vi "CreateStringParams(SubVI).vi"(1 "Show Code":bool, 2 "Line Color":string, 3 "Autoscale Mode String":string, 4 "Line Number":dbl, 5 "Cluster Graph App":T2={"Min2"=0.0, "Name2"="", "Max2"=1.0, "Min"=0.0, "Name"="", "Max"=1.0}, 6 "Cluster Line Data":T1, 7 "Cluster Mode":T3) -> (0 "params":string)   [LabVIEW 2018]
panel:
  in  "Control":string
  # "Axis Y"
  # "Axis X"
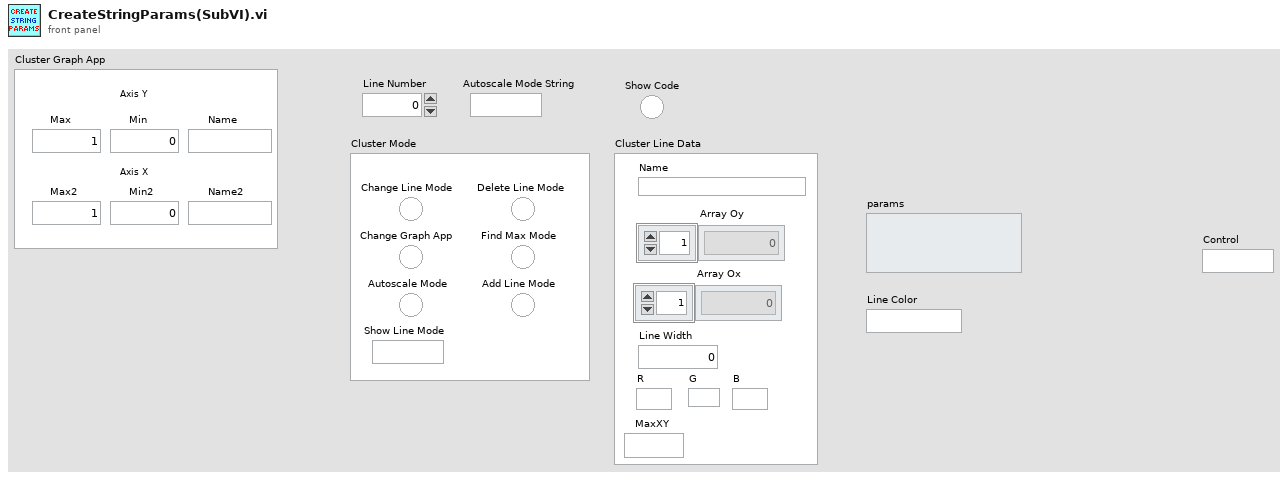
[diagram p1: front panel]
types:
  T1 = cluster{"Array Oy":dbl[], "Line Width":dbl, "Name":string, "R":string, "G":string, "B":string, "Array Ox":dbl[], "MaxXY":string}
  T2 = cluster{"Min2":dbl, "Name2":string, "Max2":dbl, "Min":dbl, "Name":string, "Max":dbl}
  T3 = cluster{"Change Line Mode":bool, "Delete Line Mode":bool, "Add Line Mode":bool, "Change Graph App":bool, "Autoscale Mode":bool, "Find Max Mode":bool, "Show Line Mode":string}
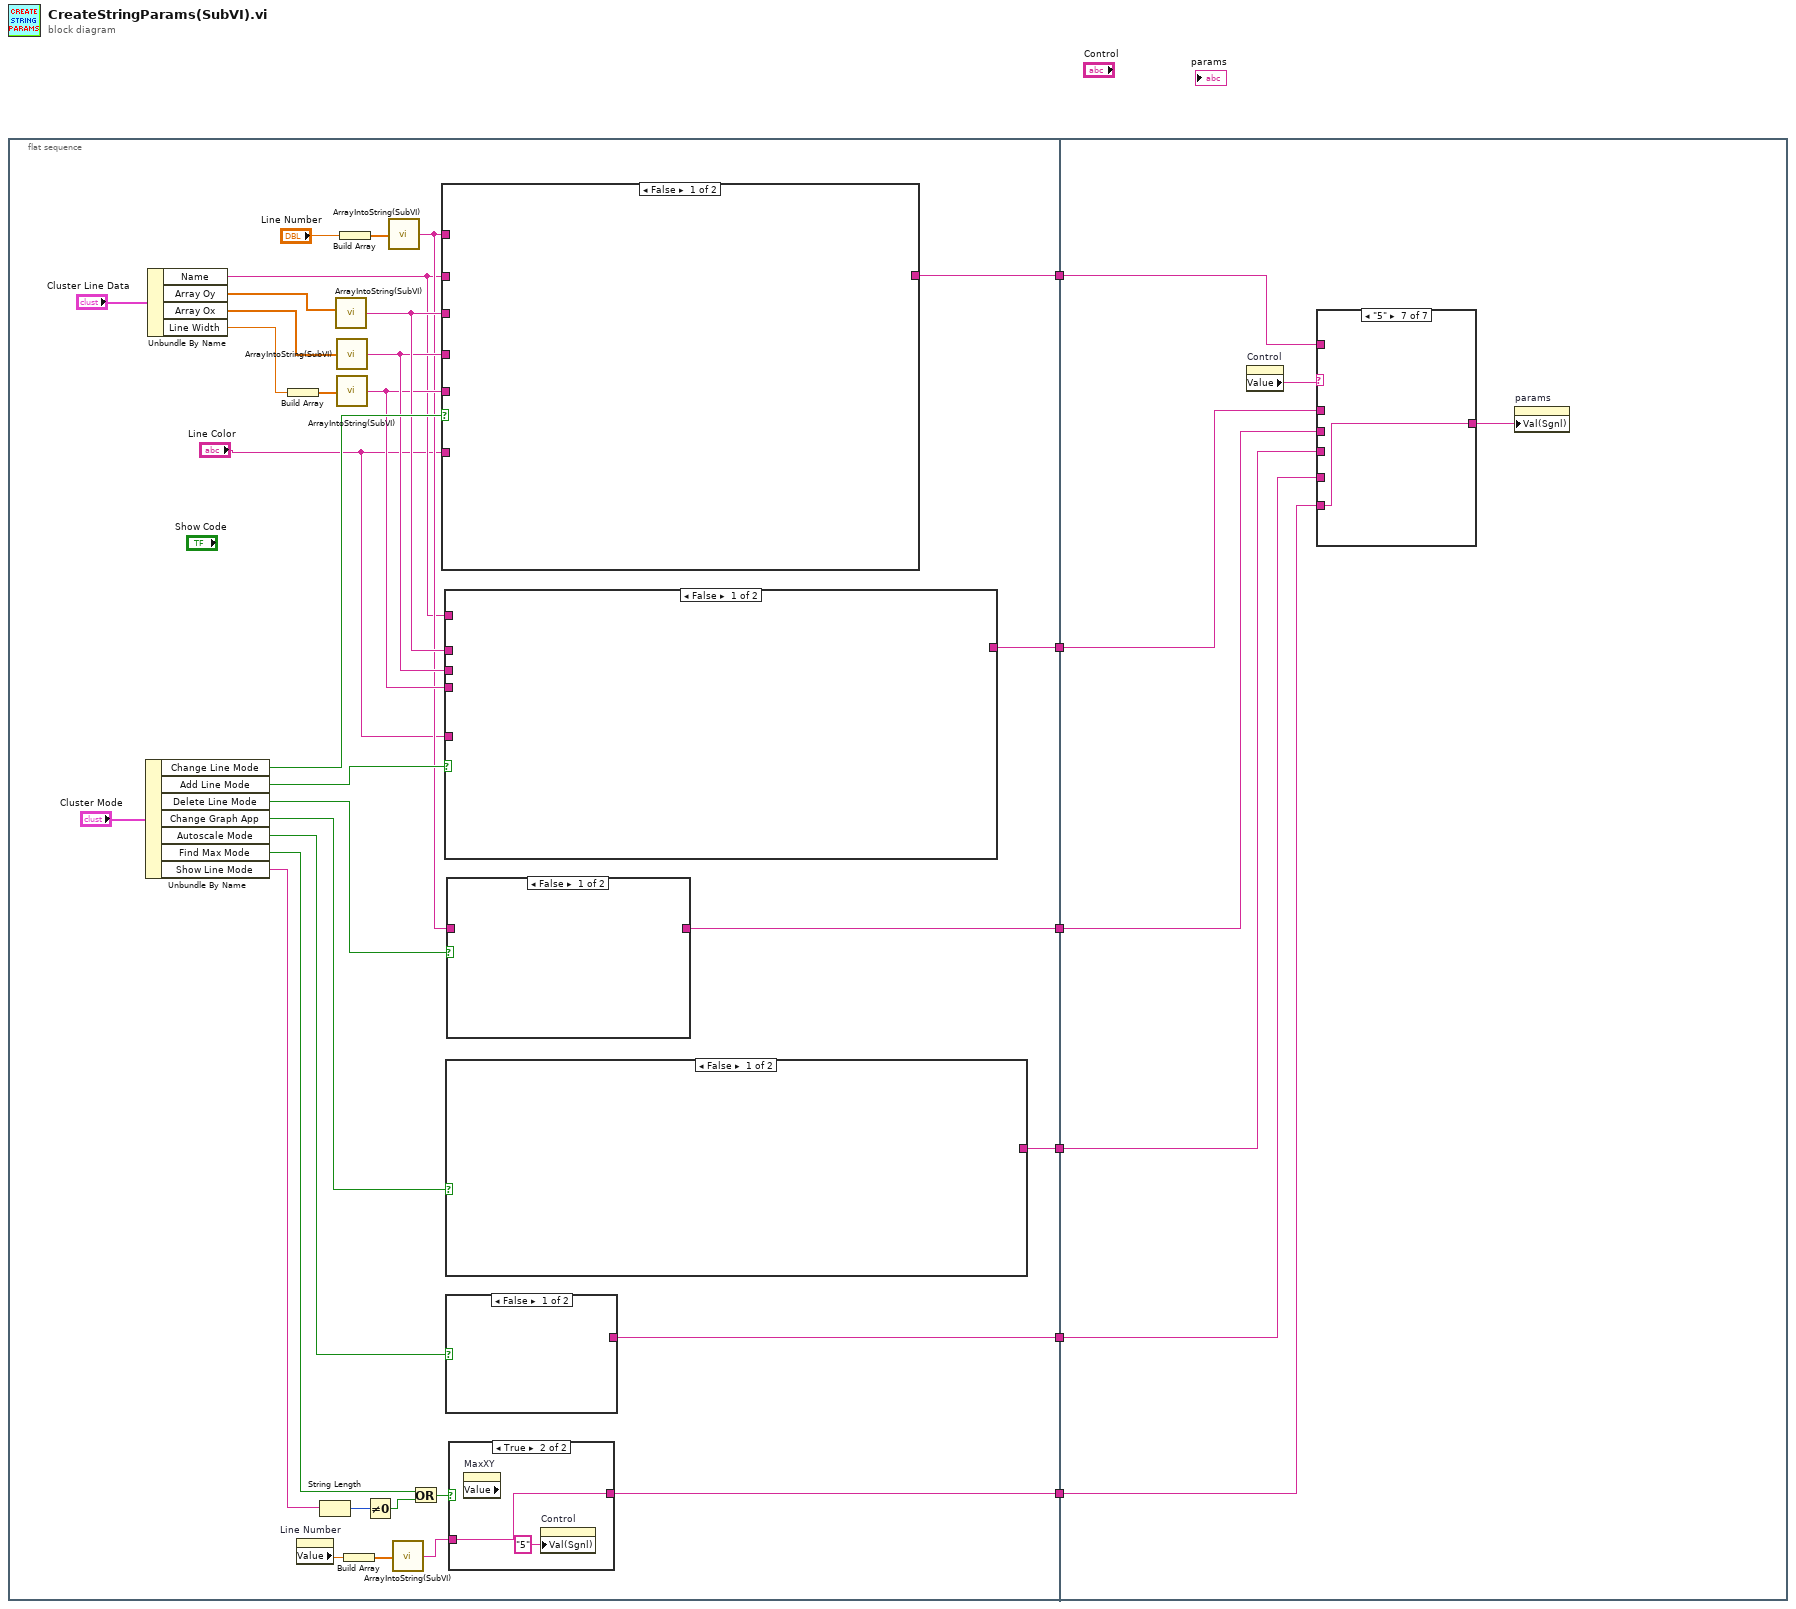
[diagram p0: block diagram]
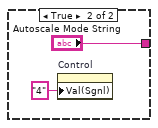
[diagram p3: hidden frame]
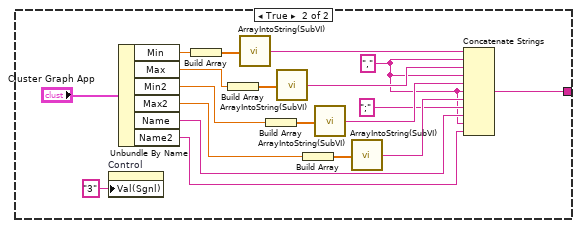
[diagram p4: hidden frame]
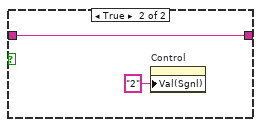
[diagram p5: hidden frame]
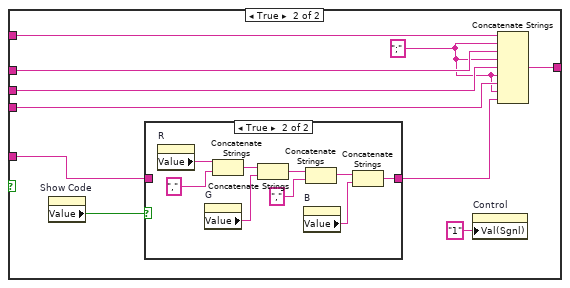
[diagram p6: hidden frame]
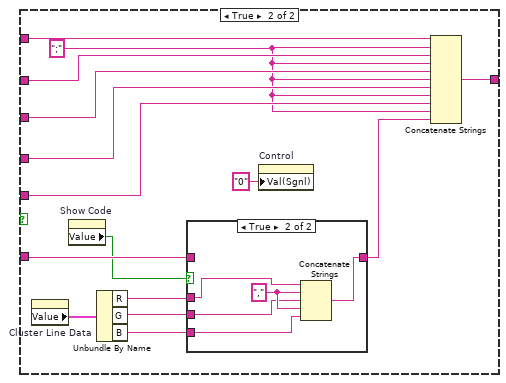
[diagram p8: hidden frame]
diagram:
  n1 = flat-sequence {
    tunnel: [w21] -> w6
    tunnel: [w20] -> w5
    tunnel: [w19] -> w4
    tunnel: [w18] -> w3
    tunnel: [w17] -> w2
    tunnel: [w16] -> w1
    tunnel: w6 -> [w112]
    tunnel: w5 -> [w111]
    tunnel: w4 -> [w110]
    tunnel: w3 -> [w109]
    tunnel: w2 -> [w108]
    tunnel: w1 -> [w107]
    frame #0 {
      n2 = Unbundle By Name("Cluster Mode") -> ("Change Line Mode"=w38:bool, "Add Line Mode"=w34:bool, "Delete Line Mode"=w30:bool, "Change Graph App"=w28:bool, "Autoscale Mode"=w22:bool, "Find Max Mode"=w10:bool, "Show Line Mode"=w7:string)
      n3 = Unbundle By Name("Cluster Line Data") -> ("Name"=w26:string, "Array Oy"=w25:dbl[], "Array Ox"=w24:dbl[], "Line Width"=w23:dbl)
      n4 = Build Array(w23) -> (w37:dbl[])
      n5 = property on="Line Number" class="DigNum (strict)"() -> ("Value"=w13:dbl)  [unwired: 2 in, 2 out]
      n6 = String Length(string=w7) -> (length=w8:i32)
      n7 = call "ArrayIntoString(SubVI).vi"("Array"=w25) -> ("Result string"=w33:string)
      n8 = call "ArrayIntoString(SubVI).vi"("Array"=w24) -> ("Result string"=w32:string)
      n9 = call "ArrayIntoString(SubVI).vi"("Array"=w37) -> ("Result string"=w31:string)
      n10 = Build Array("Line Number") -> (w36:dbl[])
      n11 = Build Array(w13) -> (w14:dbl[])
      n12 = Not Equal To 0?(x=w8) -> (x != 0?=w9:bool)
      n13 = call "ArrayIntoString(SubVI).vi"("Array"=w36) -> ("Result string"=w29:string)
      n14 = call "ArrayIntoString(SubVI).vi"("Array"=w14) -> ("Result string"=w12:string)
      n15 = Or(x=w10, y=w9) -> (x .or. y?=w11:bool)
      n16 = case shown="False" w38 {
        tunnel: w29 -> [_ w99]
        tunnel: w26 -> [_ w97]
        tunnel: w33 -> [_ w96]
        tunnel: w32 -> [_ w95]
        tunnel: w31 -> [_ w94]
        tunnel: "Line Color" -> [_ w98]
        tunnel: [_ w92] -> w21
        frame False {
        }
        frame True {
          w93 = ";" ("string")
          n17 = property on="Cluster Line Data" class="Clust (strict)"() -> ("Value"=w89:T1)  [unwired: 2 in, 2 out]
          n18 = property on="Show Code" class="Bool (strict)"() -> ("Value"=w85:bool)  [unwired: 2 in, 2 out]
          n19 = Unbundle By Name(w89) -> ("R"=w88:string, "G"=w87:string, "B"=w86:string)
          n20 = case shown="True" w85 {
            tunnel: [w100 w101] -> w91
            tunnel: w98 -> [w100 _]
            tunnel: w88 -> [_ w104]
            tunnel: w87 -> [_ w103]
            tunnel: w86 -> [_ w102]
            frame False {
            }
            frame True {
              w105 = "," ("string")
              n21 = Concatenate Strings(w104, w105, w103, w105, w102) -> (w101:string)
            }
          }
          n22 = property on="Control" class="Str"("Val(Sgnl)"="0" ("Value (Signaling)")) -> ()  [unwired: 2 in, 2 out]
          n23 = Concatenate Strings(w99, w93, w97, w93, w96, w93, w95, w93, w94, w93, w91) -> (w92:string)
        }
      }
      n24 = case shown="False" w34 {
        tunnel: w33 -> [_ w71]
        tunnel: w32 -> [_ w70]
        tunnel: w31 -> [_ w69]
        tunnel: [_ w68] -> w20
        tunnel: w26 -> [_ w74]
        tunnel: "Line Color" -> [_ w73]
        frame False {
        }
        frame True {
          w67 = ";" ("string")
          n25 = property on="Show Code" class="Bool (strict)"() -> ("Value"=w72:bool)  [unwired: 2 in, 2 out]
          n26 = case shown="True" w72 {
            tunnel: [w75 w79] -> w66
            tunnel: w73 -> [w75 _]
            frame False {
            }
            frame True {
              n27 = property on="R" class="Str"() -> ("Value"=w78:string)  [unwired: 2 in, 2 out]
              n28 = property on="G" class="Str"() -> ("Value"=w77:string)  [unwired: 2 in, 2 out]
              n29 = Concatenate Strings(w78, "," ("string")) -> (w83:string)
              n30 = Concatenate Strings(w83, w77) -> (w82:string)
              n31 = property on="B" class="Str"() -> ("Value"=w76:string)  [unwired: 2 in, 2 out]
              n32 = Concatenate Strings(w82, "," ("string")) -> (w80:string)
              n33 = Concatenate Strings(w80, w76) -> (w79:string)
            }
          }
          n34 = property on="Control" class="Str"("Val(Sgnl)"="1" ("Value (Signaling)")) -> ()  [unwired: 2 in, 2 out]
          n35 = Concatenate Strings(w74, w67, w71, w67, w70, w67, w69, w67, w66) -> (w68:string)
        }
      }
      n36 = case shown="False" w28 {
        tunnel: [_ w45] -> w18
        frame False {
        }
        frame True {
          w47 = "," ("string")
          n37 = property on="Control" class="Str"("Val(Sgnl)"="3" ("Value (Signaling)")) -> ()  [unwired: 2 in, 2 out]
          n38 = Unbundle By Name("Cluster Graph App") -> ("Min"=w60:dbl, "Max"=w58:dbl, "Min2"=w56:dbl, "Max2"=w54:dbl, "Name"=w48:string, "Name2"=w46:string)
          n39 = Build Array(w60) -> (w61:dbl[])
          n40 = Build Array(w58) -> (w59:dbl[])
          n41 = call "ArrayIntoString(SubVI).vi"("Array"=w61) -> ("Result string"=w53:string)
          n42 = Build Array(w56) -> (w57:dbl[])
          n43 = call "ArrayIntoString(SubVI).vi"("Array"=w59) -> ("Result string"=w52:string)
          n44 = Build Array(w54) -> (w55:dbl[])
          n45 = call "ArrayIntoString(SubVI).vi"("Array"=w57) -> ("Result string"=w51:string)
          n46 = call "ArrayIntoString(SubVI).vi"("Array"=w55) -> ("Result string"=w50:string)
          n47 = Concatenate Strings(w53, w47, w52, w47, w51, w47, w50, ";" ("string"), w48, w47, w46) -> (w45:string)
        }
      }
      n48 = case shown="False" w22 {
        tunnel: [_ "Autoscale Mode String"] -> w17
        frame False {
        }
        frame True {
          n49 = property on="Control" class="Str"("Val(Sgnl)"="4" ("Value (Signaling)")) -> ()  [unwired: 2 in, 2 out]
        }
      }
      n50 = case shown="False" w30 {
        tunnel: w29 -> [_ w64]
        tunnel: [_ w64] -> w19
        frame False {
        }
        frame True {
          n51 = property on="Control" class="Str"("Val(Sgnl)"="2" ("Value (Signaling)")) -> ()  [unwired: 2 in, 2 out]
        }
      }
      n52 = case shown="True" w11 {
        tunnel: [_ w40] -> w16
        tunnel: w12 -> [_ w40]
        frame False {
        }
        frame True {
          n53 = property on="MaxXY" class="Str" props=["Value"]() -> ()  [unwired: 2 in, 3 out]
          n54 = property on="Control" class="Str"("Val(Sgnl)"="5" ("Value (Signaling)")) -> ()  [unwired: 2 in, 2 out]
        }
      }
    }
    frame #1 {
      n55 = property on="Control" class="Str"() -> ("Value"=w113:string)  [unwired: 2 in, 2 out]
      n56 = case shown="\"5\"" w113 {
        tunnel: w112 -> [w114 w115 _ _ _ _ _]
        tunnel: w111 -> [_ _ w116 _ _ _ _]
        tunnel: w110 -> [_ _ _ w117 _ _ _]
        tunnel: w109 -> [_ _ _ _ w118 _ _]
        tunnel: w108 -> [_ _ _ _ _ w119 _]
        tunnel: w107 -> [_ _ _ _ _ _ w120]
        tunnel: [w114 w115 w116 w117 w118 w119 w120] -> w106
        frame "False", Default {
        }
        frame "0" {
        }
        frame "1" {
        }
        frame "2" {
        }
        frame "3" {
        }
        frame "4" {
        }
        frame "5" {
        }
      }
      n57 = property on="params" class="Str"("Val(Sgnl)"=w106) -> ()  [unwired: 2 in, 2 out]
    }
  }
